vi "Execute.vi"(8 "error in":errorcluster, 10 "Change Setpoint CMD in":refnum<class "Change Setpoint CMD.lvclass">, 11 "Object In":refnum<class>) -> (0 "error out":errorcluster, 3 "Object Out":refnum<class>)   [LabVIEW 2014, in "Humidifier Lib.lvlib" / "Change Setpoint CMD.lvclass"]
doc: "Abstract method for accomplishing the execution of a command directed to an instrument object on the wire."
uses:
  Change Setpoint CMD.lvclass
  Humidifier.lvclass
  Change Setpoint CMD.lvclass/Change Setpoint CMD.ctl
  Humidifier.lvclass/Humidifier.ctl
  Accessors/Write SP.vi
  Accessors/Read RH_.vi
  Accessors/Read Temperature Task.vi
  Accessors/Read Log Session.vi
  <vilib>/DAQmx/write.llb/DAQmx Write (Analog DBL 1Chan 1Samp).vi
  <userlib>/_Session Fwk/Session - Root.lvclass
  reusable/Session APIs/Session Log/System Log.lvclass
  reusable/General/Temperature/Temperature.lvlib
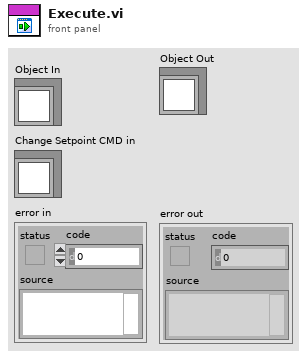
[diagram p1: front panel]
types:
  T1 = typedef "Session - Root.lvclass/Session Handle.ctl" = refnum<data-value>
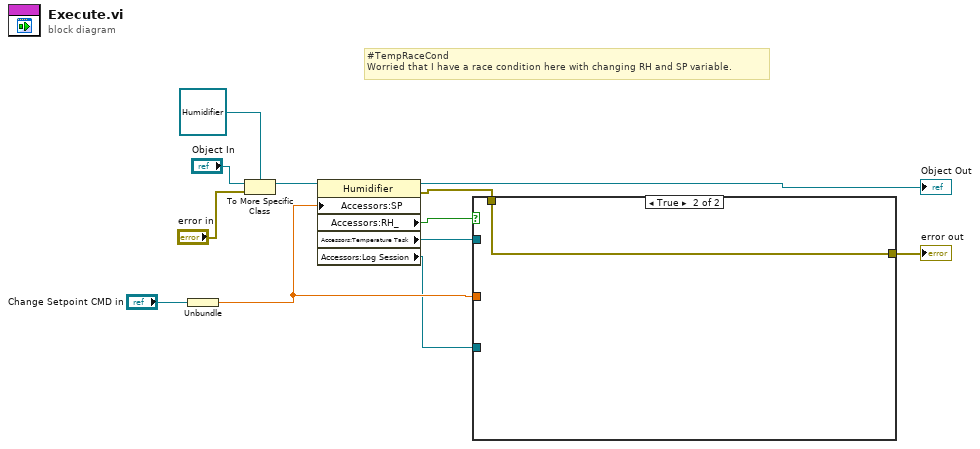
[diagram p0: block diagram]
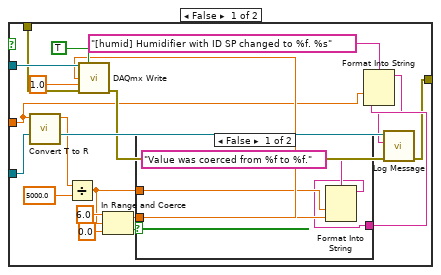
[diagram p2: hidden frame]
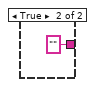
[diagram p3: hidden frame]
diagram:
  # "#TempRaceCond\nWorried that I have a race condition here with changing RH and SP variable."
  n1 = Unbundle("Change Setpoint CMD in") -> (w6:dbl)
  n2 = To More Specific Class(target class=refnum<class "Humidifier.lvclass"> refnum ("Humidifier Lib.lvlib:Humidifier"), reference="Object In", error in="error in") -> (specific class reference=w8:refnum<class "Humidifier.lvclass">)  [unwired: 1 out]
  n3 = property class="Humidifier"(reference=w8, "Accessors:SP"=w6) -> (reference out=→"Object Out":refnum<class "Humidifier.lvclass">, error out=w3:errorcluster, "Accessors:RH_"=w7:bool, "Accessors:Temperature Task"=w4:refnum<k21>, "Accessors:Log Session"=w5:T1)  [unwired: 1 in]
  n4 = case shown="True" w7 {
    tunnel: w6 -> [w16 _]
    tunnel: w5 -> [w26 _]
    tunnel: w4 -> [w30 _]
    tunnel: w3 -> [w28 w36]
    tunnel: [w13 w36] -> w1
    frame False {
      n5 = call "Convert T to R.vi"("T"=w16) -> ("R"=w24:dbl)  [unwired: 10 in]
      n6 = Divide(x=w24, y=5000.0) -> (x/y=w19:dbl)
      n7 = In Range and Coerce(upper limit=6.0, x=w19, lower limit=0.0) -> (coerced(x)=w18:dbl, In Range?=w20:bool)
      n8 = call-poly <vilib>:"DAQmx Write.vi"("task/channels in"=w30, "auto start"=TRUE, "data"=w18, "timeout"=1.0, "error in"=w28) -> ("error out"=w25:errorcluster)  [unwired: 8 in, 2 out]
      n9 = case shown="False" w20 {
        tunnel: [w31 ""] -> w15
        tunnel: w19 -> [w33 _]
        tunnel: w18 -> [w32 _]
        frame False {
          n10 = Format Into String(format string="Value was coerced from %f to %f.", w33, w32) -> (resulting string=w31:string)  [unwired: 2 in, 1 out]
        }
        frame True {
        }
      }
      n11 = Format Into String(format string="[humid] Humidifier with ID SP changed to %f. %s", w16, w15) -> (resulting string=w14:string)  [unwired: 2 in, 1 out]
      n12 = call "Log Message.vi"("error in"=w25, "MSG In"=w14, "session in"=w26) -> ("error out"=w13:errorcluster)  [unwired: 7 in, 1 out]
    }
    frame True {
    }
  }
  "error out" <- w1
